vi "Send Write Bit Field.vi"(6 "Success timeout (0 = dont wait)":i32, 7 "Message Priority (Normal)":T1=enum."Normal", 8 "error in (no error)":errorcluster, 9 "Interlock Chain":refnum<class "Interlock Chain.lvclass">, 10 "Bit Field":u16, 11 "Message Enqueuer":refnum<class "Message Enqueuer.lvclass">) -> (0 "error out":errorcluster, 1 "timed out":bool, 2 "occurrence":refnum<k4>, 3 "Message Enqueuer out":refnum<class "Message Enqueuer.lvclass">)   [LabVIEW 2015, in "cRIO-Carbondioxide.lvlib" / "CO2-Actor.lvlib" / "Write Bit Field Msg.lvclass"]
doc: "This VI sends the message to an actor."
uses:
  Write Bit Field Msg.lvclass
  <vilib>/ActorFramework/Message Enqueuer/Message Enqueuer.lvclass
  <vilib>/ActorFramework/Message Enqueuer/Message Priority.ctl
  Interlocks/Interlock Chain/Interlock Chain.lvclass
  Write Bit Field Msg.lvclass/Write Bit Field Msg.ctl
  <vilib>/ActorFramework/Message Enqueuer/Message Enqueuer.lvclass/Message Enqueuer.ctl
  <vilib>/ActorFramework/Message Priority Queue/Priority Enqueue.vi
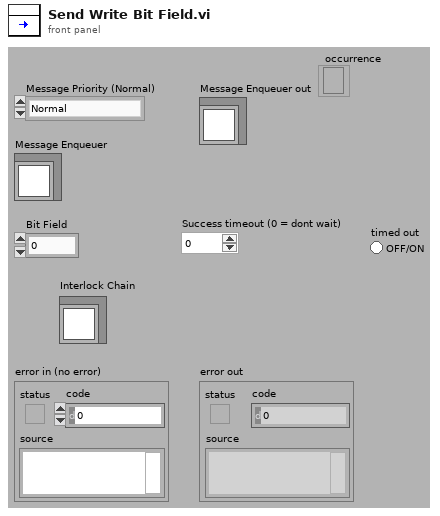
[diagram p1: front panel]
types:
  T1 = typedef "Actor Framework.lvlib/Message Enqueuer.lvclass/Message Priority.ctl" = enum16{"Low", "Normal", "High"}
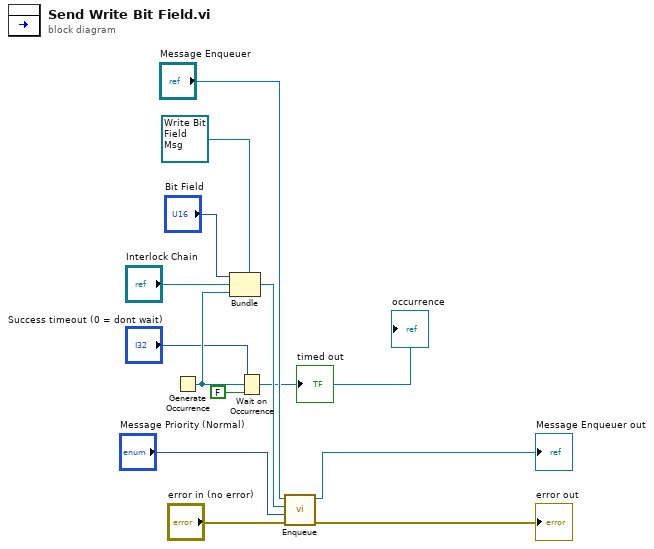
[diagram p0: block diagram]
diagram:
  n1 = Generate Occurrence() -> (w4:refnum<k4>)
  "occurrence" <- w4
  n2 = Bundle(cluster=refnum<class "Write Bit Field Msg.lvclass"> refnum ("Object"), "Bit Field", "Interlock Chain", w4) -> (w9:refnum<class "Write Bit Field Msg.lvclass">)
  n3 = Wait on Occurrence(1:FALSE ("ignore previous (T)"), 2:w4, 3:"Success timeout (0 = dont wait)") -> (0:→"timed out":bool)
  n4 = call <vilib>:"Enqueue.vi"("error in (no error)"="error in (no error)", "Message Priority (Normal)"="Message Priority (Normal)", "Message"=w9, "Message Enqueuer in"="Message Enqueuer") -> ("error out"=→"error out":errorcluster, "Message Enqueuer out"=→"Message Enqueuer out":refnum<class "Message Enqueuer.lvclass">)  [unwired: 6 in]
